vi "MS Initialization v2.vi"(6 "PID Cluster":T2={"L1 to L4 PID Cluster"={"L1 PID Gains"={"Kp"=0.005, "Kd"=0.5, "Ki"=0.0005}, "L2 PID Gains"={"Kp"=0.01, "Kd"=1.0, "Ki"=0.005}, "L3 PID Gains"={"Kp"=0.05, "Kd"=1.0, "Ki"=0.0005}, "L4 PID Gains"={"Kp"=0.1, "Kd"=0.1, "Ki"=0.0005}}, "Stage PID Cluster"={"Stage Z PID"={"Kp"=0.0005, "Kd"=0.001, "Ki"=0.0}, "Stage Y PID"={"Kp"=0.0003, "Kd"=0.01, "Ki"=0.0}, "Stage X PID"={"Kp"=0.0003, "Kd"=0.01, "Ki"=0.0}}, "OCT Z PID Gains"={"Kp"=0.0003, "Kd"=0.0001, "Ki"=0.01}}, 7 "Robot In":i32, 8 "error in":errorcluster, 10 "Prev Posit Cluster":T3={"Prev L1 to L4 Posit"=[0.0, 0.0, 0.0, 0.0], "Prev Stage Posit"=[6.0, 6.0, 6.0], "Prev OCT Z Posit"=0.0}, 11 "FPGA VI Reference In":refnum<k20>) -> (0 "error out":errorcluster, 2 "Last Posit Cluster":T1={"Last L1 to L4 Posit"=[0.0, 0.0, 0.0, 0.0], "Last Stage Posit"=[6.0, 6.0, 6.0], "Last OCT Z Posit"=0.0}, 3 "FPGA VI Reference Out":refnum<k20>)   [LabVIEW 2016]
uses:
  Subsystems/Global Variables.vi
  <vilib>/Platform/TimedLoop/XDataNode/wakeup.ctl
  <vilib>/Platform/TimedLoop/XDataNode/XDNodeRunTimeDep.lvlib
  <vilib>/Platform/TimedLoop/XDataNode/nitl_modes.ctl
  <vilib>/Platform/TimedLoop/XDataNode/timing_clust.ctl
  <vilib>/platform/TimedLoop/XDataNode/XDataNode.xnode
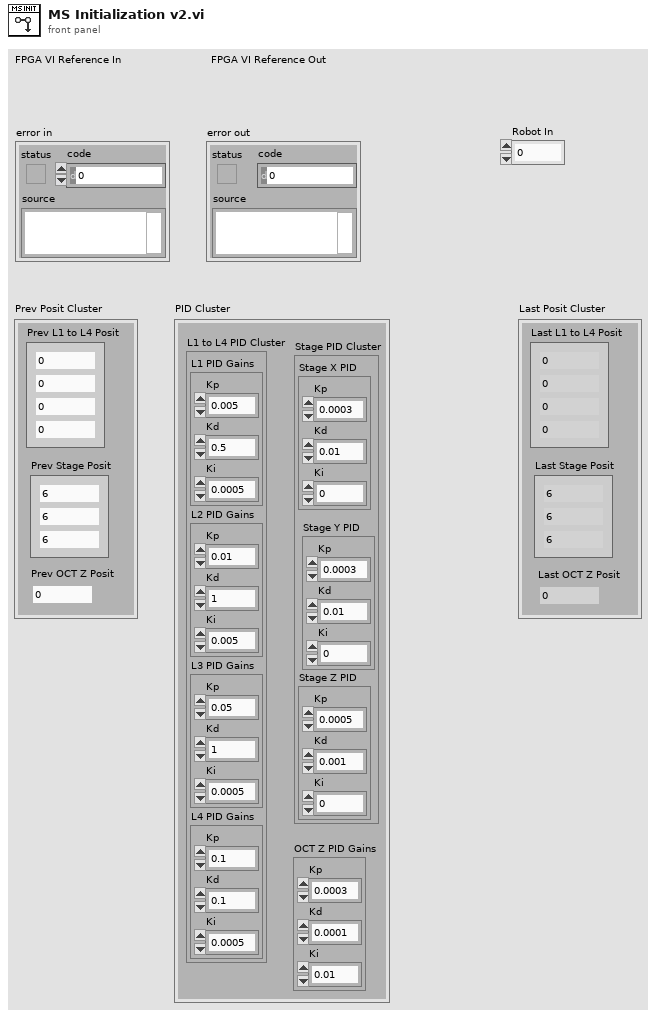
[diagram p1: front panel]
types:
  T1 = cluster{"Last L1 to L4 Posit":dbl[], "Last Stage Posit":dbl[], "Last OCT Z Posit":dbl}
  T2 = cluster{"L1 to L4 PID Cluster":cluster{"L1 PID Gains":cluster{"Kp":dbl, "Kd":dbl, "Ki":dbl}, "L2 PID Gains":cluster{"Kp":dbl, "Kd":dbl, "Ki":dbl}, "L3 PID Gains":cluster{"Kp":dbl, "Kd":dbl, "Ki":dbl}, "L4 PID Gains":cluster{"Kp":dbl, "Kd":dbl, "Ki":dbl}}, "Stage PID Cluster":cluster{"Stage Z PID":cluster{"Kp":dbl, "Kd":dbl, "Ki":dbl}, "Stage Y PID":cluster{"Kp":dbl, "Kd":dbl, "Ki":dbl}, "Stage X PID":cluster{"Kp":dbl, "Kd":dbl, "Ki":dbl}}, "OCT Z PID Gains":cluster{"Kp":dbl, "Kd":dbl, "Ki":dbl}}
  T3 = cluster{"Prev L1 to L4 Posit":dbl[], "Prev Stage Posit":dbl[], "Prev OCT Z Posit":dbl}
  T4 = typedef "XDNodeRunTimeDep.lvlib/timing_clust.ctl" = cluster{"Expected End [f-1]":u64, "Actual End [f-1]":u64, "Finished Late? [f-1]":bool, "Expected End [i-1]":u64, "Actual End [i-1]":u64, "Finished Late? [i-1]":bool, "Expected Start [i]":u64, "Actual Start [i]":u64, "Expected Start [f]":u64, "Actual Start [f]":u64, "Source Name":string, "Structure Name":string, "Period":i64, "Deadline":i64, "Offset":i64, "Start":i64, "Priority":i32, "Timeout":i32, "Mode":T5, "Wakeup Reason":T6, "Error":errorcluster, "Source Type":string, "Secondary Source Type":string, "Global End Time":u64, "Global Start Time":u64, "Frame Duration":u64, "Iteration Duration":u64, "Assigned CPU":i32, "I/O Scan Engine Mode":u32}
  T5 = typedef "XDNodeRunTimeDep.lvlib/nitl_modes.ctl" = enum32{"No Change", "Process missed periods, maintain original phase", "Discard missed periods, maintain original phase", "Process missed periods, ignore original phase", "Discard missed periods, ignore original phase"}
  T6 = typedef "XDNodeRunTimeDep.lvlib/wakeup.ctl" = enum32{"Normal", "Aborted", "Asynchronous wakeup", "Timing source error", "Timed loop error", "Timeout"}
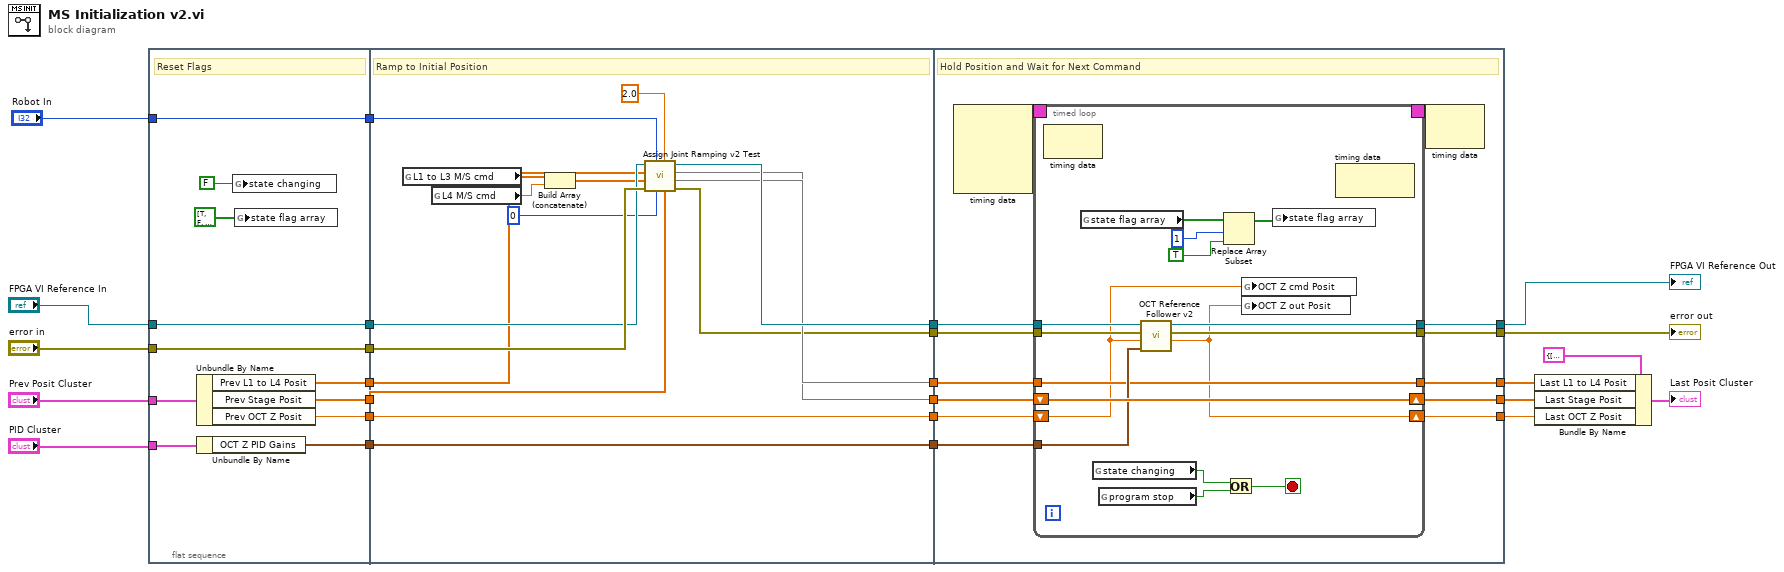
[diagram p0: block diagram]
diagram:
  n1 = flat-sequence {
    tunnel: "Prev Posit Cluster" -> [w34]
    tunnel: [w33] -> w24
    tunnel: "PID Cluster" -> [w28]
    tunnel: "error in" -> [w32]
    tunnel: [w32] -> w21
    tunnel: [w31] -> w20
    tunnel: "FPGA VI Reference In" -> [w31]
    tunnel: [w30] -> w11
    tunnel: [w29] -> w9
    tunnel: [w27] -> w7
    tunnel: "Robot In" -> [w26]
    tunnel: [w26] -> w4
    tunnel: w24 -> [w43]
    tunnel: w21 -> [w48]
    tunnel: w20 -> [w46]
    tunnel: [w51] -> w18
    tunnel: w11 -> [w38]
    tunnel: [w37] -> w10
    tunnel: w9 -> [w52]
    tunnel: [w52] -> w8
    tunnel: w7 -> [w51]
    tunnel: [w45] -> w6
    tunnel: [w40] -> w5
    tunnel: w4 -> [w47]
    tunnel: [w41] -> w2
    tunnel: w18 -> [w64]
    tunnel: [w58] -> w17
    tunnel: [w53] -> w14
    tunnel: [w63] -> w13
    tunnel: [w62] -> w12
    tunnel: [w61] -> w1
    tunnel: w10 -> [w60]
    tunnel: w8 -> [w59]
    tunnel: w6 -> [w57]
    tunnel: w5 -> [w65]
    tunnel: w2 -> [w54]
    frame #0 {
      # "Reset Flags"
      n2 = Unbundle By Name(w34) -> ("Prev L1 to L4 Posit"=w33:dbl[], "Prev Stage Posit"=w30:dbl[], "Prev OCT Z Posit"=w29:dbl)
      n3 = Unbundle By Name(w28) -> ("OCT Z PID Gains"=w27:cluster{"Kp":dbl, "Kd":dbl, "Ki":dbl})
      n4 = global write "Global Variables.vi" "state changing"(FALSE ("state changing")) -> ()
      n5 = global write "Global Variables.vi" "state flag array"(bool[] [TRUE, FALSE, FALSE, FALSE, FALSE, FALSE, FALSE, FALSE, FALSE] ("state flag array")) -> ()
    }
    frame #1 {
      # "Ramp to Initial Position"
      n6 = global read "Global Variables.vi" "L1 to L3 M/S cmd"() -> (w50:dbl[])
      n7 = global read "Global Variables.vi" "L4 M/S cmd"() -> (w49:dbl)
      n8 = Build Array (concatenate)(w50, w49) -> (w42:dbl[])
      n9 = call "Assign Joint Ramping v2 Test.vi"(4:w38, "Ramp Time [sec]"=2.0 ("Target Tool Insertion Length"), "Vac Digital Cmd"=i8 0, "Robot In"=w47, "error in"=w48, "Destination Posit Array [mm]"=w42, 10:w43, "FPGA VI Reference In"=w46) -> ("error out"=w40:errorcluster, 1:w41, 2:w37, "FPGA VI Reference Out"=w45:refnum<k20>)
    }
    frame #2 {
      # "Hold Position and Wait for Next Command"
      n10 = node-c288() -> (w56:T4)  [unwired: 4 in]
      n11 = timed-loop {
        timing: w56 -> [_]
        timing-out: [_] -> w55
        tunnel: w57 -> [w70]
        tunnel: w65 -> [w73]
        tunnel: w64 -> [w72]
        tunnel: [w71] -> w61
        shift-right: [w74] -> w63
        shift-left: w60 -> [w74]
        shift-right: [w66] -> w62
        shift-left: w59 -> [w67]
        tunnel: [w69] -> w58
        tunnel: w54 -> [w68]
        tunnel: [w68] -> w53
        stop <- w81 stop-if-true
        n12 = node-c288() -> ()  [unwired: 1 in, 1 out]
        n13 = global read "Global Variables.vi" "state flag array"() -> (w78:bool[])
        n14 = global read "Global Variables.vi" "state changing"() -> (w80:bool)
        n15 = global read "Global Variables.vi" "program stop"() -> (w79:bool)
        n16 = call "OCT Reference Follower v2.vi"("OCT Z PID Gains"=w72, "OCT  Z cmd Posit [mm]"=w67, "error in"=w73, "FPGA VI Reference In"=w70) -> ("OCT  Z out Posit [mm]"=w66:dbl, "error out"=w71:errorcluster, "FPGA VI Reference Out"=w69:refnum<k20>)  [unwired: 5 in]
        n17 = Replace Array Subset(array=w78, new element=TRUE ("new element/subarray"), index=1) -> (w77:bool[])
        n18 = Or(x=w80, y=w79) -> (x .or. y?=w81:bool)
        n19 = global write "Global Variables.vi" "OCT Z cmd Posit"(w67) -> ()
        n20 = global write "Global Variables.vi" "OCT Z out Posit"(w66) -> ()
        n21 = global write "Global Variables.vi" "state flag array"(w77) -> ()
        n22 = node-c288() -> ()  [unwired: 1 in, 1 out]
      }
      n23 = node-c288(w55) -> ()  [unwired: 1 out]
    }
  }
  n24 = Bundle By Name(cluster=T1 {"Last L1 to L4 Posit"=[0.0, 0.0, 0.0, 0.0], "Last Stage Posit"=[6.0, 6.0, 6.0], "Last OCT Z Posit"=0.0} ("Last Posit Cluster 2"), "Last L1 to L4 Posit"=w14, "Last Stage Posit"=w13, "Last OCT Z Posit"=w12) -> (→"Last Posit Cluster":T1)
  "FPGA VI Reference Out" <- w17
  "error out" <- w1
